vi "Open Standard RGB ColorProcessor.vi"(6 "Bit Depth":i32, 8 "error in (no error)":errorcluster, 9 "Color Correction Matrix":sgl[](array[numeric]), 10 "White Balance Matrix":sgl[](array[numeric]), 11 "ColorProcessorSDK reference":refnum<k24>) -> (0 "error out":errorcluster, 2 "StandardRGBColorProcessor":refnum<k24>, 3 "ColorProcessorSDK reference out":refnum<k24>)   [LabVIEW 2015]
uses:
  C:/code/ScientificCameraInterfaces/Installer/Scientific Camera Interfaces/LabVIEW/64_bit/Library_X64/Thorlabs.TSI.ColorProcessor.dll
  code/ScientificCameraInterfaces/Installer/Scientific Camera Interfaces/LabVIEW/64_bit/Library_X64/Thorlabs.TSI.ColorProcessor.dll
  C:/code/ScientificCameraInterfaces/Installer/Scientific Camera Interfaces/LabVIEW/64_bit/Library_X64/Thorlabs.TSI.ColorInterfaces.dll
  code/ScientificCameraInterfaces/Installer/Scientific Camera Interfaces/LabVIEW/64_bit/Library_X64/Thorlabs.TSI.ColorInterfaces.dll
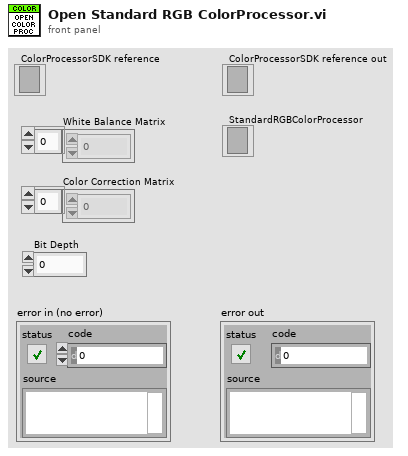
[diagram p1: front panel]
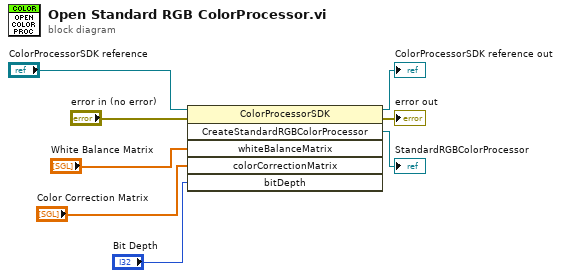
[diagram p0: block diagram]
diagram:
  n1 = invoke class="ColorProcessorSDK" method="CreateStandardRGBColorProcessor"(reference="ColorProcessorSDK reference", error in="error in (no error)", "whiteBalanceMatrix"="White Balance Matrix", "colorCorrectionMatrix"="Color Correction Matrix", "bitDepth"="Bit Depth") -> (reference out=→"ColorProcessorSDK reference out":refnum<k24>, error out=→"error out":errorcluster, "CreateStandardRGBColorProcessor"=→"StandardRGBColorProcessor":refnum<k24>)  [unwired: 1 in, 3 out]
